vi "can_send.vi"() -> ()   [LabVIEW 2009]
panel:
  in  "BTR 0":u32 caption="BTR0" format="%x"
  in  "BTR 1":u32 caption="BTR1" format="%x"
  in  "K":u16(ring)=1000 items=["10"=10, "20"=20, "50"=50, "100"=100, "125"=125, "250"=250, "500"=500, "800"=800, "1000"=1000]
  in  "Baudrate":enum32{"Standard", "Custom"}(radio)
  out "Error out":errorcluster {"code" format="%.0x"}
  in  "WriteTimeOut":u32=5000 caption="ms"
  in  "Synchronization":i32(ring)=1 items=["Synchronization"=1, "Asynchronization"=0]
  out "Transmission of MSG":string[][](table)
  in  "Data Format":enum32{"Hexadecimal", "Decimal"}(radio)
  in  "MSG_RTR":bool
  in  "CANPort":string(combo)="CAN2"
  in  "ID (HEX)":u32=2047 format="%x"
  in  "Flags":u8(ring)=4 items=["MSG_STD"=0, "MSG_EXT"=4]
  in  "Number to Write":u32=100
  in  "stop":bool
  out "NumberofWritten":u32
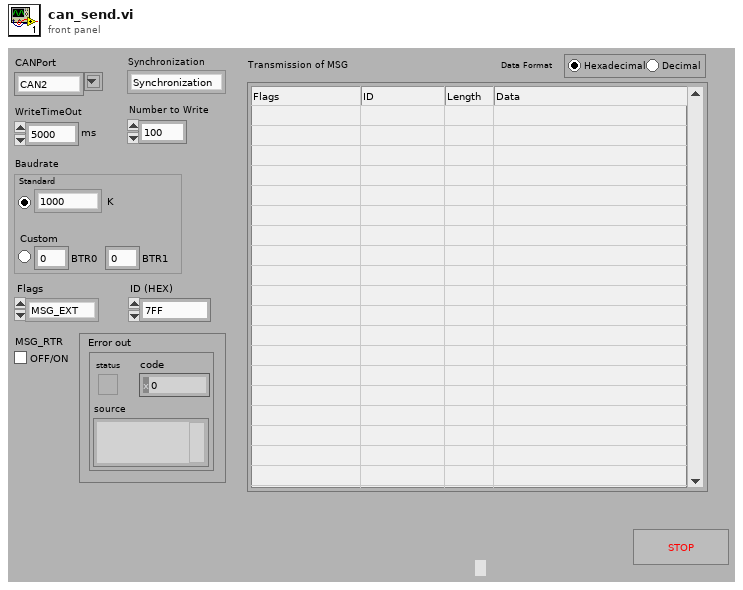
[diagram p1: front panel]
types:
  T1 = cluster{"Internal":u32, "InternalHigh":u32, "Offset":u32, "OffsetHigh":u32, "hEvent":u32}
  T2 = cluster{"Flags":u32, "ID(HEX)":u32, "Length":i16, "Data":u8[]}[]
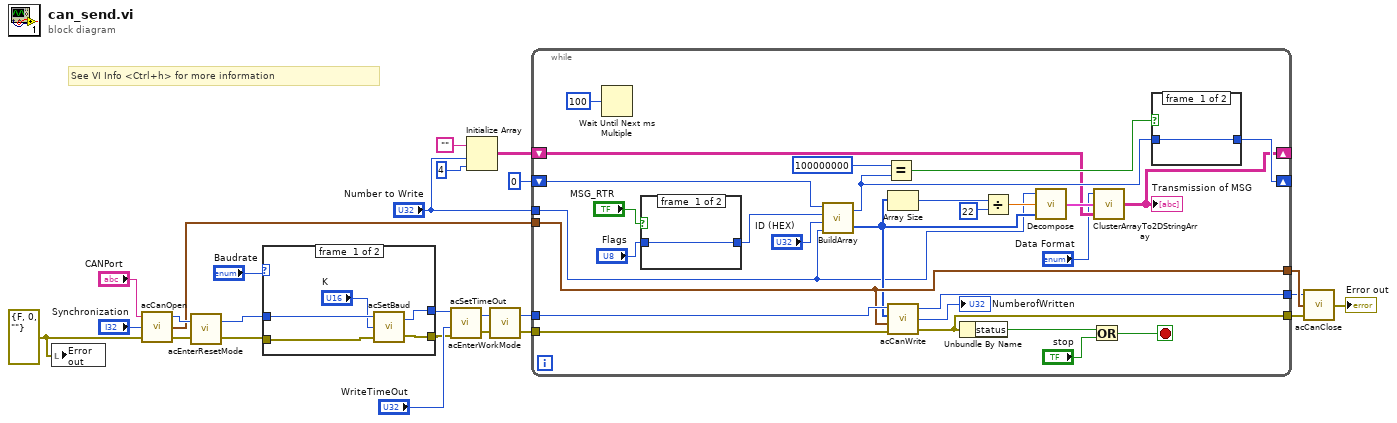
[diagram p0: block diagram]
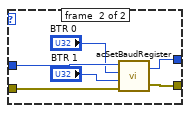
[diagram p2: hidden frame]
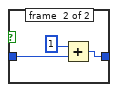
[diagram p3: hidden frame]
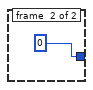
[diagram p4: hidden frame]
diagram:
  w16 = errorcluster {"status"=FALSE, "code"=0, "source"=""} ("Error in")
  # "See VI Info <Ctrl+h> for more information"
  n1 = local write "Error out"(w16) -> ()
  n2 = call "acCanOpen.vi"("Error in"=w16, "Synchronization"="Synchronization", "CANPort"="CANPort") -> ("Error out"=w22:errorcluster, "Overlapped"=w17:T1, "Handle"=w21:u32)
  n3 = call "acEnterResetMode.vi"("Error in"=w22, "Handle  in"=w21) -> ("Error out"=w3:errorcluster, "Handle out"=w2:u32)
  n4 = case shown="\"Custom\"" "Baudrate" {
    tunnel: [w29 w36] -> w4
    tunnel: [w30 w35] -> w1
    tunnel: w2 -> [w28 w33]
    tunnel: w3 -> [w27 w34]
    frame #0 {
      n5 = call "acSetBaud.vi"("Error in"=w27, "Baudrate"="K", "Handle  in"=w28) -> ("Error out"=w29:errorcluster, "Handle out"=w30:u32)
    }
    frame #1 {
      n6 = call "acSetBaudRegister.vi"("Error in"=w34, "BTR 1"="BTR 1", "BTR 0"="BTR 0", "Handle  in"=w33) -> ("Error out"=w36:errorcluster, "Handle out"=w35:u32)
    }
  }
  n7 = call "acSetTimeOut.vi"("Error in"=w4, "WriteTimeOut"="WriteTimeOut", "Handle  in"=w1) -> ("Error out"=w8:errorcluster, "Handle out"=w7:u32)  [unwired: 1 in]
  n8 = Initialize Array("", "Number to Write", 4 ("Dimension Size")) -> (w13:string[][])
  n9 = call "acEnterWorkMode.vi"("Error in"=w8, "Handle  in"=w7) -> ("Error out"=w24:errorcluster, "Handle out"=w25:u32)
  n10 = while {
    tunnel: w25 -> [w57]
    tunnel: w24 -> [w58]
    tunnel: [w61] -> w10
    tunnel: [w60] -> w9
    shift-right: [w54] -> _
    shift-left: u32 0 ("Numberto out") -> [w51]
    tunnel: w17 -> [w56]
    tunnel: [w56] -> w11
    shift-right: [w43] -> _
    shift-left: w13 -> [w44]
    tunnel: "Number to Write" -> [w42]
    stop <- w63 stop-if-true
    n11 = Wait Until Next ms Multiple(millisecond multiple=u32 100) -> ()  [unwired: 1 out]
    n12 = case shown="True" "MSG_RTR" {
      tunnel: "Flags" -> [w65 w68]
      tunnel: [w65 w66] -> w39
      frame #0 {
      }
      frame #1 {
        n13 = Add(x=u8 1, y=w68) -> (x+y=w66:u8)
      }
    }
    n14 = call "BuildArray.vi"("Number to Write"=w42, "ID"="ID (HEX)", "Flags"=w39, "Numberto in"=w51) -> ("initialized array"=w49:u8[], "Numberto out"=w53:i32)
    n15 = Equal?(x=100000000 ("y"), y=w53) -> (x = y?=w55:bool)
    n16 = Array Size(array=w49) -> (size(s)=w48:i32)
    n17 = call "acCanWrite.vi"("Error in"=w58, "Overlapped"=w56, "MSG"=w49, "Handle  in"=w57) -> ("Error out"=w61:errorcluster, "NumberOfWritten"=→"NumberofWritten":u32, "Handle out"=w60:u32)
    n18 = Unbundle By Name(w61) -> ("status"=w38:bool)
    n19 = Divide(x=w48, y=22) -> (x/y=w46:dbl)
    n20 = call "Decompose.vi"("Array"=w49, "Real"=w46, "Expect"=w42) -> ("MSG"=w45:T2)
    n21 = Or(x=w38, y="stop") -> (x .or. y?=w63:bool)
    n22 = call "ClusterArrayTo2DStringArray.vi"("Input Array"=w44, "MSG"=w45, "Data Format"="Data Format") -> ("Output Array"=w43:string[][])
    "Transmission of MSG" <- w43
    n23 = case shown="True" w55 {
      tunnel: [w69 0 ("Numberto out")] -> w54
      tunnel: w53 -> [w69 _]
      frame #0 {
      }
      frame #1 {
      }
    }
  }
  n24 = call "acCanClose.vi"("Error in"=w10, "Overlapped"=w11, "Handle  in"=w9) -> ("Error out"=→"Error out":errorcluster)
